vi "ExpDestroy.vi"(8 "error in":errorcluster, 11 "ExpID":string) -> (0 "error out":errorcluster, 3 "ExpID out":string)   [LabVIEW 2017]
uses:
  ExpGlobals.vi
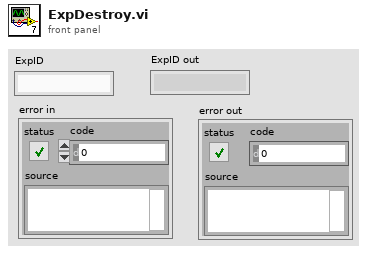
[diagram p1: front panel]
types:
  T1 = typedef "ExperimentInfo.ctl" = cluster{"ExposeInfo":T2, "ExpID":string, "ExperimentFilename":string, "Caller Keep Alive":refnum<data-value>}
  T2 = typedef "ExposeInfo.ctl" = cluster{"CSCom":refnum<k24>, "URL":string, "Events Category":string, "ID":string, "SRefID":string}
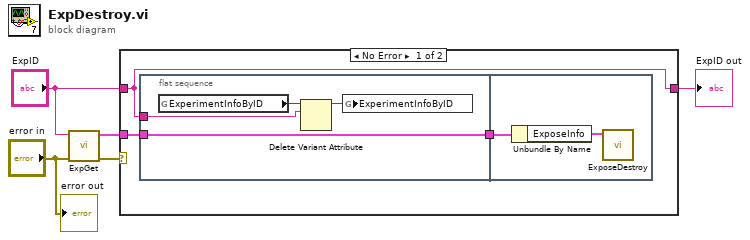
[diagram p0: block diagram]
diagram:
  n1 = call "ExpGet.vi"("error in"="error in", "ExpID"="ExpID") -> ("error out"=w5:errorcluster, "Exp Info"=w4:T1)  [unwired: 8 in]
  n2 = case shown="No Error" w5 {
    tunnel: w4 -> [w8 _]
    tunnel: "ExpID" -> [w6 w15]
    tunnel: [w6 w15] -> w1
    frame No Error {
      n3 = flat-sequence {
        tunnel: w8 -> [w12]
        tunnel: [w12] -> w7
        tunnel: w6 -> [w10]
        tunnel: w7 -> [w14]
        frame #0 {
          n4 = global read "ExpGlobals.vi" "ExperimentInfoByID"() -> (w11:variant)
          n5 = Delete Variant Attribute(6:w10, 7:w11) -> (3:w9:variant)  [unwired: 1 in, 2 out]
          n6 = global write "ExpGlobals.vi" "ExperimentInfoByID"(w9) -> ()
        }
        frame #1 {
          n7 = Unbundle By Name(w14) -> ("ExposeInfo"=w13:T2)
          n8 = call "ExposeDestroy.vi"("Expose Info"=w13) -> ()  [unwired: 9 in, 2 out]
        }
      }
    }
    frame Error {
    }
  }
  "ExpID out" <- w1
  "error out" <- "error in"
